vi "setUp.vi"(8 "error in (no error)":errorcluster, 11 "reference in":refnum<class "SLSC Switch Scripting System Tests.lvclass">=refnum) -> (0 "error out":errorcluster, 3 "reference out":refnum<class "SLSC Switch Scripting System Tests.lvclass">)   [LabVIEW 2019, in "SLSC Switch Scripting System Tests.lvclass"]
doc: "setUp runs prior to the test method during test execution. Use this method to initialize any object data required by your tests."
uses:
  SLSC Switch Scripting System Tests.lvclass
  <vilib>/addons/_JKI Toolkits/VI Tester/TestCase.llb/TestCase.lvclass
  <vilib>/NI/VeriStand Custom Device Testing Tools/VeriStandTestUtilities/VeriStandTestUtilities.lvlib
  <userlib>/_OpenG.lib/file/file.llb/Append Path to Root if Relative - Scalar__ogtk.vi
  <vilib>/NI/VeriStand Custom Device Testing Tools/VeriStandTestCase/VeriStandTestCase.lvclass
  C:/Program Files (x86)/National Instruments/LabVIEW 2019/vi.lib/addons/_JKI Toolkits/VI Tester/TestCase.llb/TestCase.lvclass
  C:/Dev/GitHub/niveristand-custom-device-testing-tools/VeriStandTestCase/VeriStandTestCase.lvclass
panel:
  in  "Minimum VeriStand Version":string="2017"
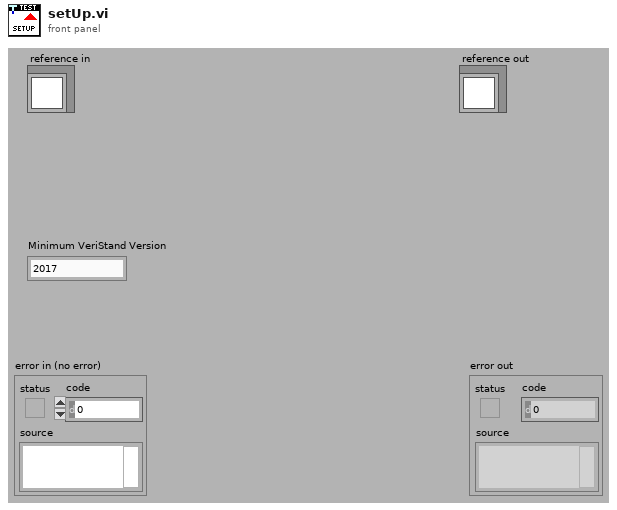
[diagram p1: front panel]
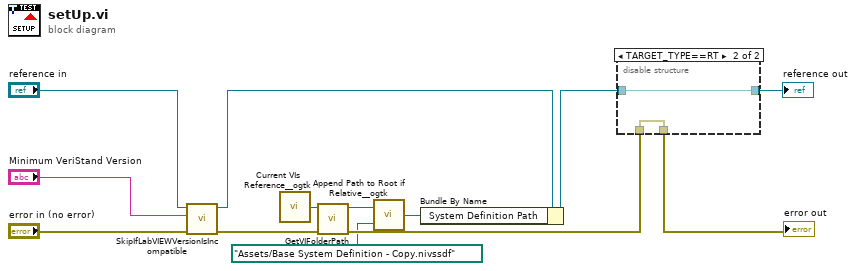
[diagram p0: block diagram]
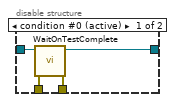
[diagram p2: hidden frame]
diagram:
  n1 = call <vilib>:"SkipIfLabVIEWVersionIsIncompatible.vi"("error in (no error)"="error in (no error)", "Minimum Version Year (2016)"="Minimum VeriStand Version", "VeriStandTestCase in"="reference in") -> ("error out"=w8:errorcluster, "VeriStandTestCase out"=w7:refnum<class "SLSC Switch Scripting System Tests.lvclass">)  [unwired: 6 in, 1 out]
  n2 = call <userlib>:"Current VIs Reference__ogtk.vi"() -> ("Current VI's reference"=w4:refnum<vi>)  [unwired: 5 in]
  n3 = call <vilib>:"GetVIFolderPath.vi"("error in (no error)"=w8, "VI Reference in"=w4) -> ("error out"=w6:errorcluster, "VI Folder Path out"=w3:path)  [unwired: 8 in]
  n4 = call-poly <userlib>:"Append Path to Root if Relative__ogtk.vi"("Absolute or Relative Path"=path "Assets/Base System Definition - Copy.nivssdf", "Root Path"=w3) -> ("Absolute or Appended Path"=w1:path)
  n5 = Bundle By Name(cluster=w7, "System Definition Path"=w1) -> (w5:refnum<class "SLSC Switch Scripting System Tests.lvclass">)
  n6 = disable-structure shown="TARGET_TYPE==RT" {
    disable-tunnel: w6 -> [w17 w18]
    disable-tunnel: [w16 w18] -> w13
    disable-tunnel: [w15 w19] -> w12
    disable-tunnel: w5 -> [w14 w19]
    frame condition #0 (active) {
      n7 = call <vilib>:"WaitOnTestComplete.vi"("error in (no error)"=w17, "TestCase in"=w14) -> ("error out"=w16:errorcluster, "TestCase out"=w15:refnum<class "SLSC Switch Scripting System Tests.lvclass">)  [unwired: 8 in]
    }
    frame condition #1 {
    }
  }
  "error out" <- w13
  "reference out" <- w12
